vi "2012_07_25_local.vi"(0 "MC Power Data In":waveform(dbl)[](array[waveform]), 1 "Motor Power Data In":waveform(dbl)[](array[waveform]), 5 "Power \nSetting":i8(slide) min=0 max=100 step=10 scale=0.0..100.0, 7 "On/Off Control":T1(ring), 9 "Motor":i16=1, 11 "Error In":errorcluster, 12 "Fine Data In":dbl[][][](array[numeric])) -> (6 "Power \nSetting":i8(slide) min=0 max=100 step=10 scale=0.0..100.0, 14 "Fine Data Out":dbl[][][](array[numeric]), 15 "Errors":errorcluster)   [LabVIEW 2011]
uses:
  <vilib>/express/express arith-compare/Formula/XNode/ExpressFormulaBlockNode.xnode
  <vilib>/Analysis/NI_AALBase.lvlib
panel:
  in  "coarse path":path=path "Durability/coarse.lvm"
  in  "fine path":path=path "Durability/fine.lvm"
  out "Efficiency (%)":dbl format="%#.4f"
  in  "Manual Save\nFine Event":bool
  in  "Motor1 ID":string
  in  "User":string
  in  "Comments (cleared when written to file)":string
  out "Elapsed Time (s)":string caption="Elapsed Time Text"
  out "Start Time":string caption="Start Time Text"
  in  "Motor Failure\n(click to reset)":bool
  out "Coarse":bool caption="Time has Elapsed"
  out "Fine":bool caption="Time has Elapsed"
  out "Temps":dynamicdata(graph) caption="Signal Out"
  out "Power Graph":dynamicdata(graph) caption="Collected Signals"
  out "RPM":dynamicdata(graph) caption="Collected Signals"
  out "Motor RPM":dbl format="%#.0f"
  out "Power to Motor (W)":dbl format="%#.4f"
  out "Power to MC (W)":dbl format="%#.4f"
  out "Supply Voltage (V)":dbl format="%#.4f"
  in  "Run":bool
  out "Motor Temp (F)":dbl format="%.1f"
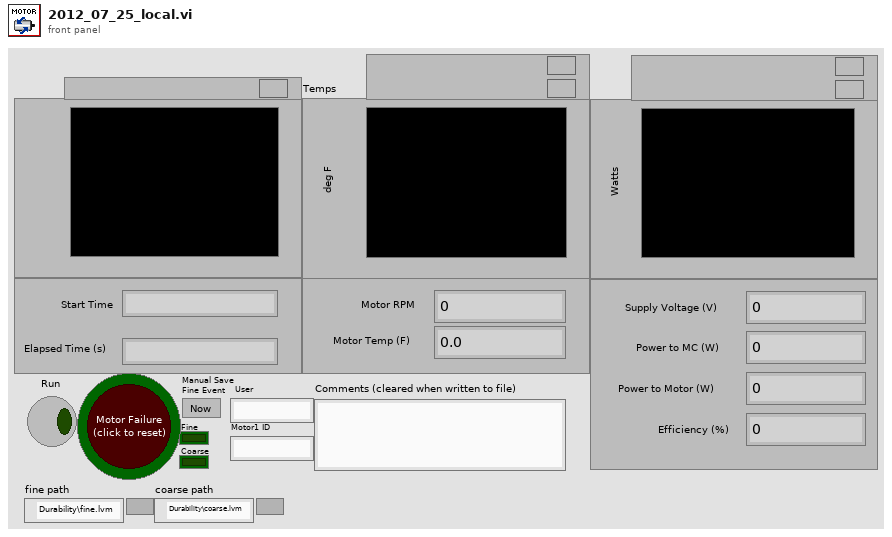
[diagram p1: front panel]
types:
  T1 = enum8{"Enabled", "Disabled", "Disabled and Grayed Out"}
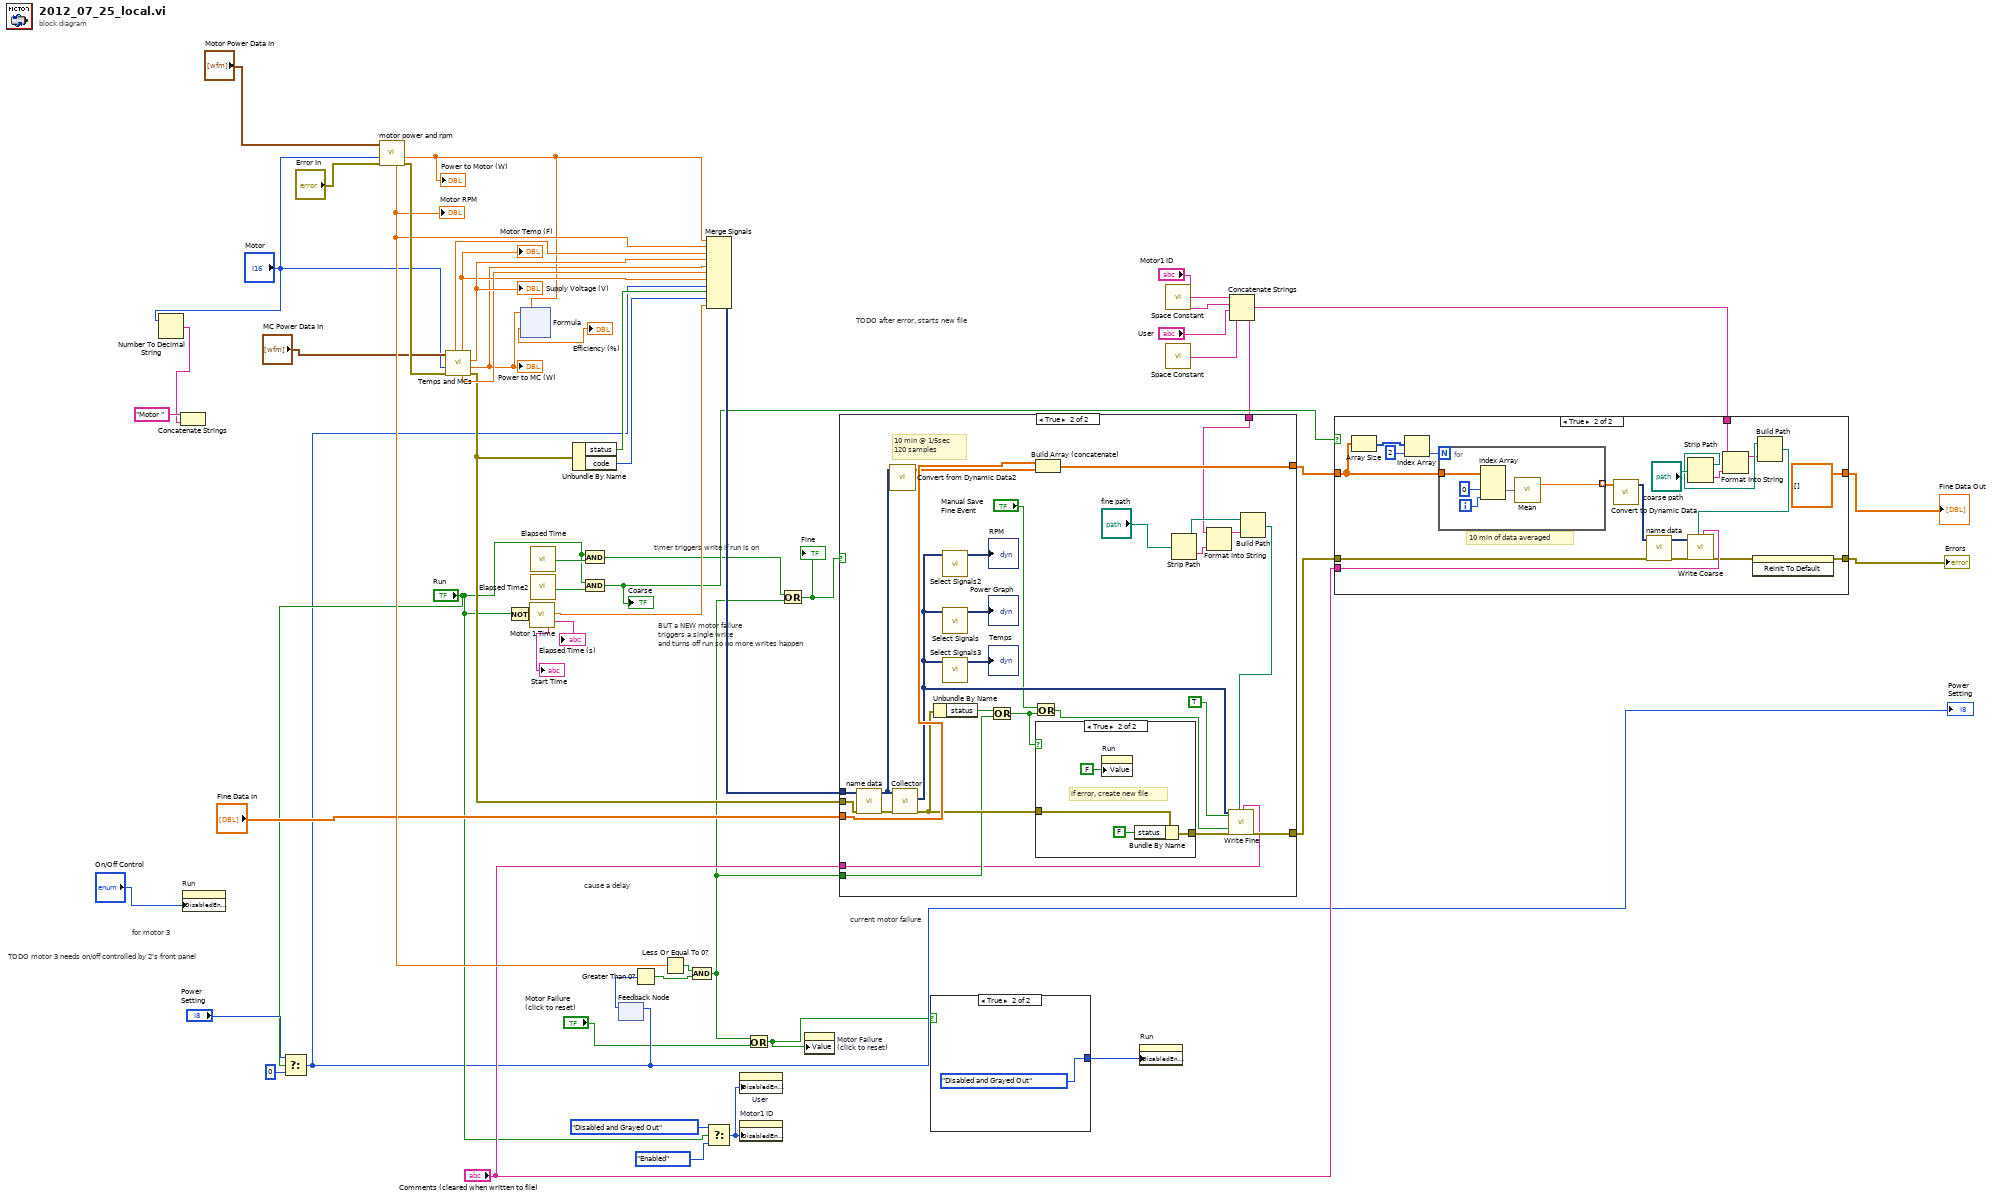
[diagram p0: block diagram]
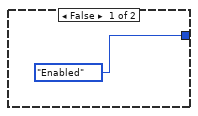
[diagram p2: hidden frame]
diagram:
  # "TODO motor 3 needs on/off controlled by 2's front panel"
  # "for motor 3"
  # "cause a delay"
  # "TODO after error, starts new file"
  # "timer triggers write if run is on"
  # "BUT a NEW motor failure\ntriggers a single write\nand turns off run so no more writes happen"
  # "current motor failure"
  n1 = Number To Decimal String(number="Motor") -> (decimal integer string=w14:string)  [unwired: 1 in]
  n2 = Concatenate Strings("Motor ", w14) -> ()  [unwired: 1 out]
  n3 = property on="Run" class="Bool (strict)"("DisabledEnum"="On/Off Control") -> ()  [unwired: 2 in, 2 out]
  n4 = Select(t="Power \nSetting", s="Run", f=i8 0) -> (s? t:f=w6:i8)
  "Power \nSetting" <- w6
  n5 = call "motor power and rpm.vi"("error in (no error)"="Error In", "Motor"="Motor", "data"="Motor Power Data In") -> ("error out"=w54:errorcluster, "Power"=w31:dbl, "RPM"=w44:dbl)  [unwired: 4 in, 2 out]
  "Motor RPM" <- w44
  "Power to Motor (W)" <- w31
  n6 = call "Temps and MCs.vi"("error in (no error)"=w54, "Motor"="Motor", "data"="MC Power Data In") -> ("error out"=w19:errorcluster, "Power 1"=w30:dbl, "Voltage 1"=w49:dbl, "Tank Temp"=w48:dbl, "Motor Temp"=w47:dbl, "Current 1"=w53:dbl)  [unwired: 3 in]
  "Motor Temp (F)" <- w47
  "Supply Voltage (V)" <- w49
  "Power to MC (W)" <- w30
  n7 = Not(x="Run") -> (.not. x?=w39:bool)
  n8 = xnode ("Formula")("MC PWR"=w30, "M PWR"=w31) -> ("Result"=→"Efficiency (%)":dbl)  [unwired: 1 in, 1 out]
  n9 = call "Motor 1 Time"("Reset"=w39) -> ("Start Time Text"=→"Start Time":string, "Elapsed Time (s)"=w38:dbl, "Elapsed Time Text"=→"Elapsed Time (s)":string)  [unwired: 11 in, 5 out]
  n10 = call "Elapsed Time"() -> ("Time has Elapsed"=w32:bool)  [unwired: 12 in, 7 out]
  n11 = call "Elapsed Time2"() -> ("Time has Elapsed"=w34:bool)  [unwired: 12 in, 7 out]
  n12 = Unbundle By Name(w19) -> ("status"=w52:bool, "code"=w51:i32)
  n13 = And(x="Run", y=w32) -> (x .and. y?=w4:bool)
  n14 = And(x="Run", y=w34) -> (x .and. y?=w33:bool)
  "Coarse" <- w33
  n15 = feedback-in #1(w6) -> ()
  n16 = feedback #1() -> (w5:i8)  [unwired: 1 in]
  n17 = Greater Than 0?(x=w5) -> (x > 0?=w42:bool)
  n18 = Less Or Equal To 0?(x=w44) -> (x <= 0?=w43:bool)
  n19 = And(x=w43, y=w42) -> (x .and. y?=w3:bool)
  n20 = Merge Signals(w31, w44, w53, w49, w30, w48, w47, w6, w52, w51, w38) -> (w50:dynamicdata)
  n21 = Select(t=T1."Disabled and Grayed Out" ("Disabled"), s="Run", f=T1."Enabled" ("Disabled")) -> (s? t:f=w35:T1)
  n22 = property on="User" class="Str"("DisabledEnum"=w35) -> ()  [unwired: 2 in, 2 out]
  n23 = property on="Motor1 ID" class="Str"("DisabledEnum"=w35) -> ()  [unwired: 2 in, 2 out]
  n24 = Or(x=w3, y="Motor Failure\n(click to reset)") -> (x .or. y?=w1:bool)
  n25 = Or(x=w4, y=w3) -> (x .or. y?=w7:bool)
  "Fine" <- w7
  n26 = property on="Motor Failure\n(click to reset)" class="Bool (strict)"("Value"=w1) -> ()  [unwired: 2 in, 2 out]
  n27 = case shown="True" w1 {
    tunnel: [T1."Enabled" ("Disabled") T1."Disabled and Grayed Out" ("Disabled")] -> w9
    frame False {
    }
    frame True {
    }
  }
  n28 = property on="Run" class="Bool (strict)"("DisabledEnum"=w9) -> ()  [unwired: 2 in, 2 out]
  n29 = call <vilib>:"Space Constant.vi"() -> ("String"=w25:string)
  n30 = call <vilib>:"Space Constant.vi"() -> ("String"=w23:string)
  n31 = Concatenate Strings("Motor1 ID", w25, "User", w23) -> (w22:string)
  n32 = case shown="True" w7 {
    tunnel: w50 -> [_ w81]
    tunnel: w19 -> [w58 w78]
    tunnel: [w58 w73] -> w8
    tunnel: [w57 w85] -> w45
    tunnel: "Fine Data In" -> [w57 w84]
    tunnel: w3 -> [_ w70]
    tunnel: "Comments (cleared when written to file)" -> [_ w69]
    tunnel: w22 -> [_ w62]
    frame False {
    }
    frame True {
      # "10 min @ 1/5sec\n120 samples"
      n33 = call "name data.vi"("error in (no error)"=w78, "Dynamic Data"=w81) -> ("error out"=w79:errorcluster, "Output"=w80:dynamicdata)  [unwired: 8 in]
      n34 = call "Convert from Dynamic Data2"("Dynamic Data Type"=w80) -> ("Array"=w83:dbl[][])  [unwired: 3 in]
      n35 = call "Collector"("error in (no error)"=w79, "Signals"=w80) -> ("error out"=w71:errorcluster, "Collected Signals"=w74:dynamicdata)  [unwired: 8 in]
      n36 = Unbundle By Name(w71) -> ("status"=w60:bool)
      n37 = call "Select Signals2"("Signals"=w74) -> ("Signal Out"=→"RPM":dynamicdata)  [unwired: 9 in, 1 out]
      n38 = call "Select Signals"("Signals"=w74) -> ("Signal Out"=→"Power Graph":dynamicdata)  [unwired: 9 in, 1 out]
      n39 = call "Select Signals3"("Signals"=w74) -> ("Signal Out"=→"Temps":dynamicdata)  [unwired: 9 in, 1 out]
      n40 = Or(x=w60, y=w70) -> (x .or. y?=w59:bool)
      n41 = Or(x="Manual Save\nFine Event", y=w59) -> (x .or. y?=w68:bool)
      n42 = Build Array (concatenate)(w84, w83) -> (w85:dbl[][][])
      n43 = case shown="True" w59 {
        tunnel: [w86 w90] -> w72
        tunnel: w71 -> [w86 w89]
        frame False {
        }
        frame True {
          # "if error, create new file"
          n44 = property on="Run" class="Bool (strict)"("Value"=FALSE ("Manual Start")) -> ()  [unwired: 2 in, 2 out]
          n45 = Bundle By Name(cluster=w89, "status"=FALSE) -> (w90:errorcluster)
        }
      }
      n46 = Strip Path(path="fine path") -> (stripped path=w65:path, name=w61:string)
      n47 = Format Into String(initial string=w62, w61) -> (resulting string=w66:string)  [unwired: 2 in, 1 out]
      n48 = Build Path(base path=w65, name or relative path=w66) -> (appended path=w63:path)
      n49 = call "Write Fine"("Signals"=w74, "Reset"=TRUE, "new_file"=w68, "error in (no error)"=w72, "Filename"=w63, "Comment"=w69) -> ("error out"=w73:errorcluster)  [unwired: 11 in, 2 out]
    }
  }
  n50 = case shown="True" w33 {
    tunnel: w45 -> [w92 w111]
    tunnel: [w92 dbl[][][] []] -> w46
    tunnel: w8 -> [w91 w103]
    tunnel: [w91 w99] -> w28
    tunnel: "Comments (cleared when written to file)" -> [_ w101]
    tunnel: w22 -> [_ w94]
    frame False {
    }
    frame True {
      # "10 min of data averaged"
      n51 = Array Size(array=w111) -> (size(s)=w107:i32[])
      n52 = Index Array(array=w107, index=2) -> (element=w108:i32)
      n53 = for {
        N: w108 -> [_]
        tunnel: w111 -> [w116]
        tunnel: [w112] -> w106 mode=indexing
        i -> [w115]
        n54 = Index Array(array=w116, index (dim 1)=0 ("disabled index (row)"), index (dim 2)=w115) -> (element=w114:dbl[])  [unwired: 1 in]
        n55 = call <vilib>:"Mean.vi"("X"=w114) -> ("mean"=w112:dbl)  [unwired: 1 out]
      }
      n56 = call "Convert to Dynamic Data"("Array"=w106) -> ("Dynamic Data Type"=w105:dynamicdata)  [unwired: 3 in]
      n57 = call "name data.vi"("error in (no error)"=w103, "Dynamic Data"=w105) -> ("error out"=w102:errorcluster, "Output"=w104:dynamicdata)  [unwired: 8 in]
      n58 = Strip Path(path="coarse path") -> (stripped path=w97:path, name=w95:string)
      n59 = Format Into String(initial string=w94, w95) -> (resulting string=w96:string)  [unwired: 2 in, 1 out]
      n60 = Build Path(base path=w97, name or relative path=w96) -> (appended path=w93:path)
      n61 = call "Write Coarse"("Signals"=w104, "error in (no error)"=w102, "Filename"=w93, "Comment"=w101) -> ("error out"=w100:errorcluster)  [unwired: 13 in, 2 out]
      n62 = invoke on="Comments (cleared when written to file)" class="Str" method="Reinit To Default"(error in=w100) -> (error out=w99:errorcluster)  [unwired: 2 in, 2 out]
    }
  }
  "Errors" <- w28
  "Fine Data Out" <- w46
